vi "MTM2_getSample_tangentForce.vi"(8 "error in (no error)":errorcluster, 11 "tangentForce_Ctl":T1={"private_rcvStamp"=0.0, "lutGravity[6]"=[0.0, 0.0, 0.0, 0.0, 0.0, 0.0], "lutTemperature[6]"=[0.0, 0.0, 0.0, 0.0, 0.0, 0.0], "applied[6]"=[0.0, 0.0, 0.0, 0.0, 0.0, 0.0], "measured[6]"=[0.0, 0.0, 0.0, 0.0, 0.0, 0.0], "hardpointCorrection[6]"=[0.0, 0.0, 0.0, 0.0, 0.0, 0.0]}) -> (0 "error out":errorcluster, 2 "function return":i32, 3 "tangentForce_Ctl out":T1)   [LabVIEW 2018, in "SALLV_MTM2.lvlib"]
doc: "int MTM2_shm_getSample_tangentForceLV(MTM2_tangentForceLV *tangentForce_Ctl );"
uses:
  DataTypes/tangentForce.ctl
  SALLV_MTM2.lvlib
  SALLV_MTM2.so
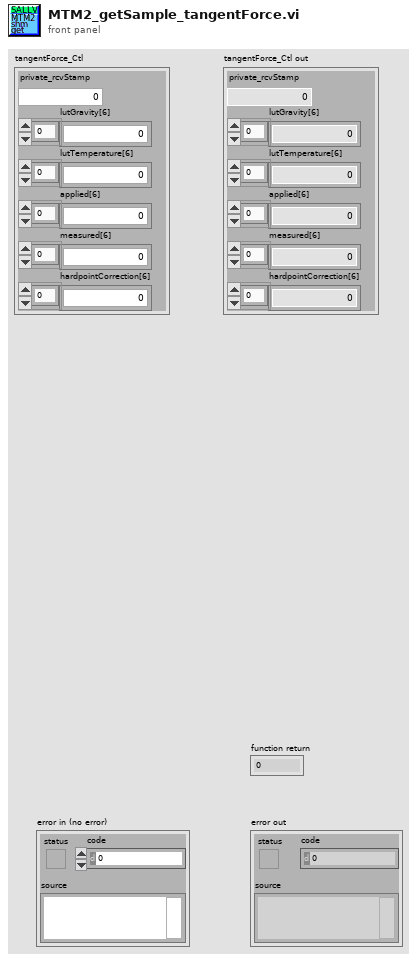
[diagram p1: front panel]
types:
  T1 = typedef "SALLV_MTM2.lvlib/tangentForce.ctl" = cluster{"private_rcvStamp":dbl, "lutGravity[6]":dbl[], "lutTemperature[6]":dbl[], "applied[6]":dbl[], "measured[6]":dbl[], "hardpointCorrection[6]":dbl[]}
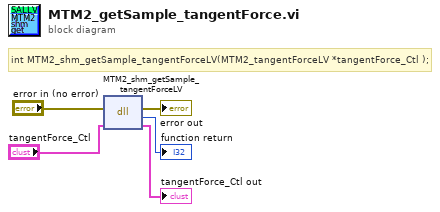
[diagram p0: block diagram]
diagram:
  # "int MTM2_shm_getSample_tangentForceLV(MTM2_tangentForceLV *tangentForce_Ctl );"
  n1 = dll-call lib="home/ttsai/Documents/salLabviewApi/SALLV_MTM2/SALLV_MTM2.*" fn="MTM2_shm_getSample_tangentForceLV"(error in="error in (no error)", "tangentForce_Ctl"="tangentForce_Ctl") -> (error out=→"error out":errorcluster, →"function return":i32, "tangentForce_Ctl"=→"tangentForce_Ctl out":T1)  [unwired: 2 in, 1 out]
